vi "Get Object Refs from Node.vi"(8 "error in (no error)":errorcluster, 11 "Data Value Reference in":T1) -> (0 "error out":errorcluster, 3 "references":T2)   [LabVIEW 2013, in "OPC UA editor node.lvclass"]
doc: "Gets the reference to the engine and a generic Module Editor Node reference from the node we have. This will be used for operations in the UI."
uses:
  OPC UA editor node.lvclass
  <vilib>/NI/DCAF Table API/Table Manager/object ref.ctl
  <vilib>/NI/DCAF/Tag Editor Core/Configuration Editor/Classes/Engine Parent/Engine Parent Editor Node.lvclass
  <vilib>/NI/DCAF/Tag Editor Core/Configuration Editor/Classes/Module editor node/module editor node.lvclass
  <vilib>/NI/Configuration Framework/Node/NodeRef.ctl
  <vilib>/NI/Configuration Framework/Node/NISE_CEF_Node.lvclass
  <vilib>/NI/DCAF Table API/Table Manager/Table Manager.lvclass
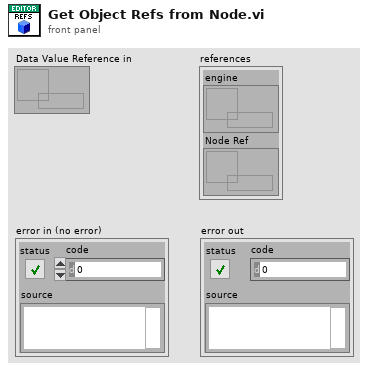
[diagram p1: front panel]
types:
  T1 = typedef "NISE_CEF_Node.lvclass/NodeRef.ctl" = refnum<data-value>
  T2 = typedef "Table Manager.lvlib/Table Manager.lvclass/object ref.ctl" = cluster{"engine":refnum<data-value>, "Node Ref":refnum<data-value>}
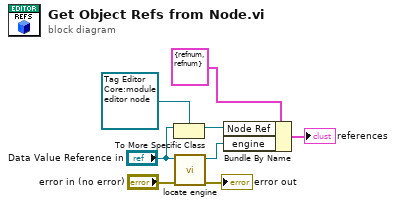
[diagram p0: block diagram]
diagram:
  n1 = To More Specific Class(target class=refnum<data-value> refnum ("data value reference"), reference="Data Value Reference in") -> (specific class reference=w6:refnum<data-value>)  [unwired: 1 in, 1 out]
  n2 = call <vilib>:"locate engine.vi"("error in"="error in (no error)", "component"="Data Value Reference in") -> ("error out"=→"error out":errorcluster, "engine"=w2:refnum<data-value>)  [unwired: 8 in]
  n3 = Bundle By Name(cluster=T2 {"engine"=refnum, "Node Ref"=refnum} ("references"), "Node Ref"=w6, "engine"=w2) -> (→"references":T2)
